vi "Run.vi"(8 "error in (no error)":errorcluster, 11 "LUnit Inheriting Test Case In":refnum<class "LUnit Inheriting Test Case.lvclass">) -> (0 "error out":errorcluster, 1 "Done?":bool, 2 "Results":T1[](array[typedef]), 3 "LUnit Inheriting Test Case Out":refnum<class "LUnit Inheriting Test Case.lvclass">)   [LabVIEW 2020, in "LUnit Inheriting Test Case.lvclass"]
doc: "Execute test and return result."
uses:
  LUnit Inheriting Test Case.lvclass
  Core/Result/Result.ctl
  Core/Result/Status.ctl
  Core/Result/Type.ctl
  LUnit Inheriting Test Case.lvclass/LUnit Inheriting Test Case.ctl
  LUnit Test Case/LUnit Test Case.lvclass
  Core/Result/Result.lvlib
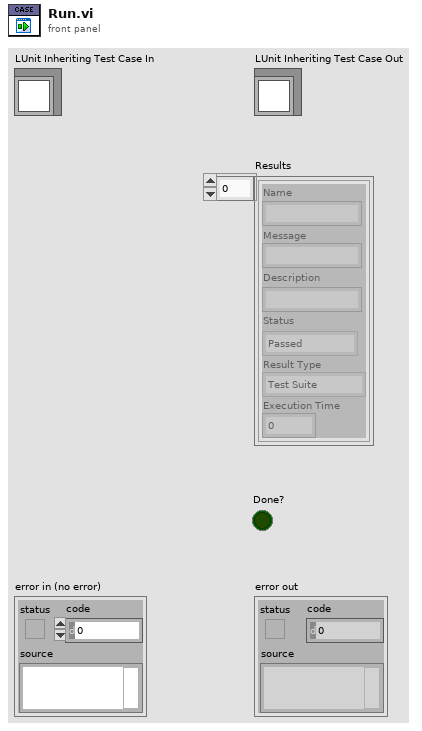
[diagram p1: front panel]
types:
  T1 = typedef "Result.lvlib/Result.ctl" = cluster{"Name":string, "Message":string, "Description":string, "Status":T2, "Result Type":T3, "Execution Time":dbl}
  T2 = typedef "Result.lvlib/Status.ctl" = enum16{"", "Passed", "Failed", "Error", "Skipped", "Setup Error", "Broken", "Teardown Error"}
  T3 = typedef "Result.lvlib/Type.ctl" = enum16{"Test Case", "Test Suite", "Test Run", "Pass", "Fail", "Skip", "Pass if", "Fail if", "Pass if Error", "Fail if Error", "Pass if Equal", "Fail if Equal"}
  T4 = typedef "Semaphore RefNum" = refnum<k1>
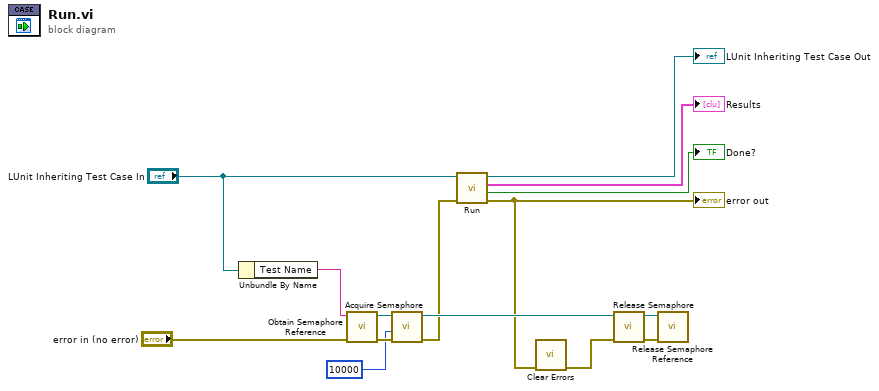
[diagram p0: block diagram]
diagram:
  n1 = Unbundle By Name("LUnit Inheriting Test Case In") -> ("Test Name"=w1:string)
  n2 = call <vilib>:"Obtain Semaphore Reference.vi"("error in (no error)"="error in (no error)", "name (unnamed)"=w1) -> ("error out"=w11:errorcluster, "semaphore"=w12:T4)  [unwired: 3 in, 1 out]
  n3 = call <vilib>:"Acquire Semaphore.vi"("error in (no error)"=w11, "ms timeout (-1)"=10000, "semaphore"=w12) -> ("error out"=w5:errorcluster, "semaphore out"=w10:T4)  [unwired: 2 in, 1 out]
  n4 = call-parent "Run.vi"("error in (no error)"=w5, "LUnit Test Case In"="LUnit Inheriting Test Case In") -> ("error out"=w3:errorcluster, "Done?"=→"Done?":bool, "Results"=→"Results":T1[], "LUnit Test Case Out"=→"LUnit Inheriting Test Case Out":refnum<class "LUnit Inheriting Test Case.lvclass">)  [unwired: 6 in]
  "error out" <- w3
  n5 = call <vilib>:"Clear Errors.vi"("error in (no error)"=w3) -> ("error out"=w7:errorcluster)  [unwired: 5 in, 1 out]
  n6 = call <vilib>:"Release Semaphore.vi"("error in (no error)"=w7, "semaphore"=w10) -> ("error out"=w8:errorcluster, "semaphore out"=w9:T4)  [unwired: 4 in]
  n7 = call <vilib>:"Release Semaphore Reference.vi"("error in (no error)"=w8, "semaphore"=w9) -> ()  [unwired: 8 in, 2 out]
